vi "Range to TC Span.vi"(8 "Floating Point Position (2)":i32=2, 9 "Scaling? (False)":bool, 10 "Range and Span":T1={"Thermocouple Type (0 : R)"=0, "Enable Span (False)"=FALSE, "Lower Span (0.0)"=0.0, "Upper Span (1760.0)"=1760.0, "Bias (0)"=0.0} {"Thermocouple Type (0 : R)" items=["R", "S", "B", "K", "K-H", "E", "J", "T", "N", "W", "L", "U", "WRe3-25", "PLATINEL", "PR40-20", "KpvsAu7Fe", "NiNiMo", "WWRe26", "N14", "XK"]; "Bias (0)" format="%_5g"; "Upper Span (1760.0)" min=-99999.0 max=99999.0 step=1.0 format="%_5g"; "Lower Span (0.0)" min=-99999.0 max=99999.0 step=0.1 format="%.1g"}, 11 "Temp. Unit (0: C)":enum16{"C", "F"}(ring)) -> (1 "Bias":i32, 2 "Upper Span":i32, 3 "Lower Span":i32)   [LabVIEW 2020, in "Yokogawa GX Series.lvlib"]
doc: "This VI gets the TC span value from the range."
uses:
  <instrlib>/Yokogawa GX Series/Yokogawa GX Series.lvlib
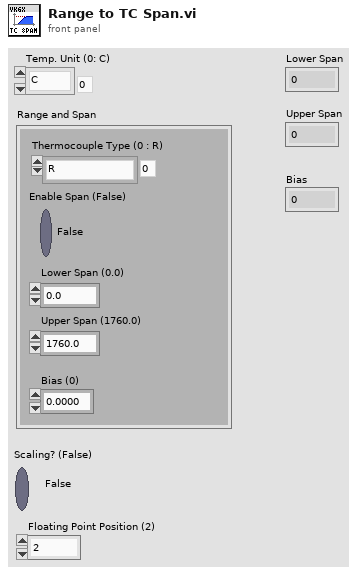
[diagram p1: front panel]
types:
  T1 = cluster{"Thermocouple Type (0 : R)":i32, "Enable Span (False)":bool, "Lower Span (0.0)":dbl, "Upper Span (1760.0)":dbl, "Bias (0)":dbl}
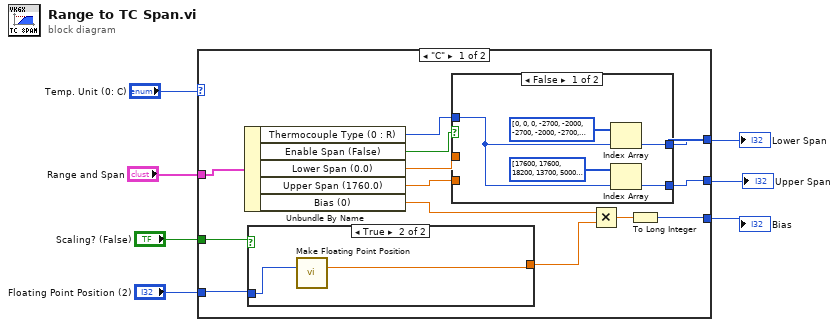
[diagram p0: block diagram]
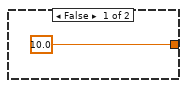
[diagram p2: hidden frame]
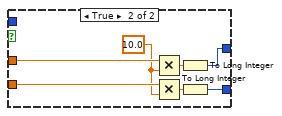
[diagram p3: hidden frame]
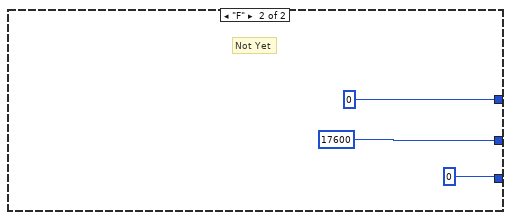
[diagram p4: hidden frame]
diagram:
  n1 = case shown="\"C\"" "Temp. Unit (0: C)" {
    tunnel: [w20 0] -> w5
    tunnel: [w19 17600] -> w6
    tunnel: "Range and Span" -> [w18 _]
    tunnel: [w13 0] -> w3
    tunnel: "Scaling? (False)" -> [w9 _]
    tunnel: "Floating Point Position (2)" -> [w8 _]
    frame "C" {
      n2 = Unbundle By Name(w18) -> ("Thermocouple Type (0 : R)"=w17:i32, "Enable Span (False)"=w16:bool, "Lower Span (0.0)"=w15:dbl, "Upper Span (1760.0)"=w14:dbl, "Bias (0)"=w10:dbl)
      n3 = case shown="True" w9 {
        tunnel: [10.0 w22] -> w11
        tunnel: w8 -> [_ w23]
        frame False {
        }
        frame True {
          n4 = call <instrlib>:"Make Floating Point Position.vi"("Floating Point Position (2)"=w23) -> ("Times"=w22:dbl)  [unwired: 14 in]
        }
      }
      n5 = case shown="False" w16 {
        tunnel: w17 -> [w28 _]
        tunnel: w15 -> [_ w34]
        tunnel: w14 -> [_ w33]
        tunnel: [w27 w31] -> w20
        tunnel: [w26 w30] -> w19
        frame False {
          n6 = Index Array(array=i32[] [0, 0, 0, -2700, -2000, -2700, -2000, -2700, -2700, 0, -2000, -2000, 0, 0, 0, 0, 0, 0, 0, -2000], index=w28) -> (element=w27:i32)
          n7 = Index Array(array=i32[] [17600, 17600, 18200, 13700, 5000, 8000, 11000, 4000, 13000, 23150, 9000, 4000, 23200, 13950, 19000, 3000, 13100, 23200, 13000, 6000], index=w28) -> (element=w26:i32)
        }
        frame True {
          w29 = 10.0
          n8 = Multiply(x=w34, y=w29) -> (x*y=w35:dbl)
          n9 = Multiply(x=w33, y=w29) -> (x*y=w32:dbl)
          n10 = To Long Integer(number=w35) -> (32bit integer=w31:i32)
          n11 = To Long Integer(number=w32) -> (32bit integer=w30:i32)
        }
      }
      n12 = Multiply(x=w10, y=w11) -> (x*y=w12:dbl)
      n13 = To Long Integer(number=w12) -> (32bit integer=w13:i32)
    }
    frame "F" {
      # "Not Yet"
    }
  }
  "Upper Span" <- w6
  "Lower Span" <- w5
  "Bias" <- w3
